vi "ByRef Parallel Read.vi"   [LabVIEW 2012]
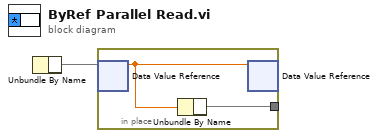
[diagram p0: block diagram]
diagram:
  n1 = Unbundle By Name() -> (w1)  [unwired: 1 in]
  n2 = in-place {
    in-place-border: [w2] -> _
    n3 = in-place-dvr #1(w1) -> (w3:dbl)  [unwired: 1 out]
    n4 = Unbundle By Name(w3) -> (w2)
    n5 = in-place-dvr #1(w3) -> ()  [unwired: 2 out]
  }
